vi "Configure Steps.vi"(8 "error in (no error)":errorcluster, 11 "Harmonics in":refnum<class "Harmonics.lvclass">) -> (0 "error out":errorcluster, 3 "Harmonics out":refnum<class "Harmonics.lvclass">)   [LabVIEW 2018, in "Harmonics.lvlib" / "Harmonics.lvclass"]
uses:
  Harmonics.lvclass
  Harmonics.lvclass/Harmonics.ctl
  Read Harmonics.vi
  Read Harmonics Pins.vi
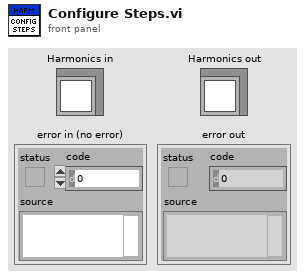
[diagram p1: front panel]
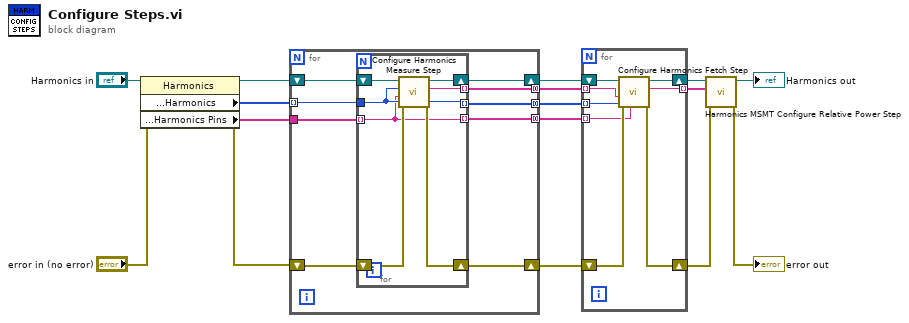
[diagram p0: block diagram]
diagram:
  n1 = property class="Harmonics"(reference="Harmonics in", error in="error in (no error)") -> (reference out=w15:refnum<class "Harmonics.lvclass">, error out=w16:errorcluster, "Protected Methods:Harmonics"=w11:i8[], "Protected Methods:Harmonics Pins"=w4:string[])
  n2 = for {
    shift-right: [w25] -> w13
    shift-left: w16 -> [w23]
    shift-right: [w24] -> w14
    shift-left: w15 -> [w21]
    tunnel: w11 -> [w20] mode=indexing
    tunnel: [w22] -> w3 mode=concatenating
    tunnel: w4 -> [w19]
    tunnel: [w18] -> w2 mode=concatenating
    tunnel: [w17] -> w1 mode=concatenating
    n3 = for {
      tunnel: [w29] -> w22 mode=indexing
      tunnel: w20 -> [w27]
      shift-right: [w32] -> w25
      shift-left: w23 -> [w30]
      shift-right: [w31] -> w24
      shift-left: w21 -> [w28]
      tunnel: w19 -> [w26] mode=indexing
      tunnel: [w27] -> w18 mode=indexing
      tunnel: [w26] -> w17 mode=indexing
      n4 = call "Configure Harmonics Measure Step.vi"("error in (no error)"=w30, "SA Pin"=w26, "Harmonic Order"=w27, "Harmonics in"=w28) -> ("error out"=w32:errorcluster, "Result Name"=w29:string, "Harmonics out"=w31:refnum<class "Harmonics.lvclass">)  [unwired: 5 in]
    }
  }
  n5 = for {
    shift-right: [w37] -> w9
    shift-left: w14 -> [w38]
    shift-right: [w39] -> w12
    shift-left: w13 -> [w40]
    tunnel: [w36] -> w8 mode=indexing
    tunnel: w3 -> [w35] mode=indexing
    tunnel: w2 -> [w34] mode=indexing
    tunnel: w1 -> [w33] mode=indexing
    n6 = call "Configure Harmonics Fetch Step.vi"("SA Pin"=w33, "error in (no error)"=w40, "Result Name"=w35, "Harmonic Order"=w34, "Harmonics in"=w38) -> ("error out"=w39:errorcluster, "Exported Data Location"=w36:string, "Harmonics out"=w37:refnum<class "Harmonics.lvclass">)  [unwired: 4 in]
  }
  n7 = call "Harmonics MSMT Configure Relative Power Step.vi"("error in (no error)"=w12, "Export Data Locations"=w8, "Harmonics in"=w9) -> ("error out"=→"error out":errorcluster, "Harmonics out"=→"Harmonics out":refnum<class "Harmonics.lvclass">)  [unwired: 7 in]
